vi "Lab Panel V4.88.vi"() -> ()   [LabVIEW 2013] (continued)
                    n2522 = Bundle("FAIL LAB02-2"=w4756, "SIG LAB02-2"=w4766, "TEMP START LAB02-2"=w4765, "DISP LAB02-2"=w4762, "SET LAB02-2"=w4761, "TDMS LAB02-2"=w4764) -> (w4751:T35)  [unwired: 1 in]
                    n2523 = call "sub vi - cycle&temp fail v7.vi"("Amps Lo?"=w4763, "Input Cluster"=w4751, "SELECT"=w4760, "Amps Hi?"=w4759, "Result In"=w4753) -> ("(FAIL) out"=w4755:cluster{"FAIL LO":dbl, "FAIL HI":dbl}, "(DISP) out"=w4758:T4, "T-RISE"=w4752:cluster{"T-RISE (L)":dbl, "T-RISE (N)":dbl}, "Result Out"=w4754:bool, "file error"=w4757:errorcluster)  [unwired: 10 in]
                    n2524 = local write "TEMP RISE LAB02-2"(w4752) -> ()
                    n2525 = local write "FAIL LAB02-2"(w4755) -> ()
                    n2526 = local write "DISP LAB02-2"(w4758) -> ()
                    n2527 = local write "RESULT LAB02-2"(w4754) -> ()
                    n2528 = local write "data file error"(w4757) -> ()
                  }
                }
              }
              frame #4 {
                # "LAB03-1"
                n2529 = case shown="True" w4768 {
                  tunnel: w4770 -> [_ w4783]
                  tunnel: w4767 -> [_ w4780]
                  tunnel: w4769 -> [_ w4779]
                  frame False {
                  }
                  frame True {
                    n2530 = local read "TEMP START LAB03-1"() -> (w4785:cluster{"TL":dbl, "TN":dbl})
                    n2531 = local read "FAIL LAB03-1"() -> (w4776:cluster{"LO":dbl, "HI":dbl})
                    n2532 = local read "TDMS LAB03-1"() -> (w4784:refnum<k34>)
                    n2533 = local read "SET LAB03-1"() -> (w4781:T5)
                    n2534 = local read "DISP LAB03-1"() -> (w4782:T4)
                    n2535 = local read "SIG LAB03-1"() -> (w4786:T2)
                    n2536 = local read "RESULT LAB03-1"() -> (w4773:bool)
                    n2537 = Bundle("FAIL LAB03-1"=w4776, "SIG LAB03-1"=w4786, "TEMP START LAB03-1"=w4785, "DISP LAB03-1"=w4782, "SET LAB03-1"=w4781, "TDMS LAB03-1"=w4784) -> (w4771:T36)  [unwired: 1 in]
                    n2538 = call "sub vi - cycle&temp fail v7.vi"("Amps Lo?"=w4783, "Input Cluster"=w4771, "SELECT"=w4780, "Amps Hi?"=w4779, "Result In"=w4773) -> ("(FAIL) out"=w4775:cluster{"FAIL LO":dbl, "FAIL HI":dbl}, "(DISP) out"=w4778:T4, "T-RISE"=w4772:cluster{"T-RISE (L)":dbl, "T-RISE (N)":dbl}, "Result Out"=w4774:bool, "file error"=w4777:errorcluster)  [unwired: 10 in]
                    n2539 = local write "TEMP RISE LAB03-1"(w4772) -> ()
                    n2540 = local write "FAIL LAB03-1"(w4775) -> ()
                    n2541 = local write "DISP LAB03-1"(w4778) -> ()
                    n2542 = local write "RESULT LAB03-1"(w4774) -> ()
                    n2543 = local write "data file error"(w4777) -> ()
                  }
                }
              }
              frame #5 {
                # "LAB03-2"
                n2544 = case shown="True" w4788 {
                  tunnel: w4790 -> [_ w4803]
                  tunnel: w4787 -> [_ w4800]
                  tunnel: w4789 -> [_ w4799]
                  frame False {
                  }
                  frame True {
                    n2545 = local read "TEMP START LAB03-2"() -> (w4805:cluster{"TL":dbl, "TN":dbl})
                    n2546 = local read "FAIL LAB03-2"() -> (w4796:cluster{"LO":dbl, "HI":dbl})
                    n2547 = local read "TDMS LAB03-2"() -> (w4804:refnum<k34>)
                    n2548 = local read "SET LAB03-2"() -> (w4801:T5)
                    n2549 = local read "DISP LAB03-2"() -> (w4802:T4)
                    n2550 = local read "RESULT LAB03-2"() -> (w4793:bool)
                    n2551 = local read "SIG LAB03-2"() -> (w4806:T2)
                    n2552 = Bundle("FAIL LAB03-2"=w4796, "SIG LAB03-2"=w4806, "TEMP START LAB03-2"=w4805, "DISP LAB03-2"=w4802, "SET LAB03-2"=w4801, "TDMS LAB03-2"=w4804) -> (w4791:T37)  [unwired: 1 in]
                    n2553 = call "sub vi - cycle&temp fail v7.vi"("Amps Lo?"=w4803, "Input Cluster"=w4791, "SELECT"=w4800, "Amps Hi?"=w4799, "Result In"=w4793) -> ("(FAIL) out"=w4795:cluster{"FAIL LO":dbl, "FAIL HI":dbl}, "(DISP) out"=w4798:T4, "T-RISE"=w4792:cluster{"T-RISE (L)":dbl, "T-RISE (N)":dbl}, "Result Out"=w4794:bool, "file error"=w4797:errorcluster)  [unwired: 10 in]
                    n2554 = local write "FAIL LAB03-2"(w4795) -> ()
                    n2555 = local write "TEMP RISE LAB03-2"(w4792) -> ()
                    n2556 = local write "DISP LAB03-2"(w4798) -> ()
                    n2557 = local write "RESULT LAB03-2"(w4794) -> ()
                    n2558 = local write "data file error"(w4797) -> ()
                  }
                }
              }
              frame #6 {
                # "LAB04-1"
                n2559 = case shown="True" w4808 {
                  tunnel: w4810 -> [_ w4823]
                  tunnel: w4807 -> [_ w4820]
                  tunnel: w4809 -> [_ w4819]
                  frame False {
                  }
                  frame True {
                    n2560 = local read "TEMP START LAB04-1"() -> (w4825:cluster{"TL":dbl, "TN":dbl})
                    n2561 = local read "FAIL LAB04-1"() -> (w4816:cluster{"LO":dbl, "HI":dbl})
                    n2562 = local read "TDMS LAB04-1"() -> (w4824:refnum<k34>)
                    n2563 = local read "SET LAB04-1"() -> (w4821:T5)
                    n2564 = local read "DISP LAB04-1"() -> (w4822:T4)
                    n2565 = local read "SIG LAB04-1"() -> (w4826:T2)
                    n2566 = local read "RESULT LAB04-1"() -> (w4813:bool)
                    n2567 = Bundle("FAIL LAB04-1"=w4816, "SIG LAB04-1"=w4826, "TEMP START LAB04-1"=w4825, "DISP LAB04-1"=w4822, "SET LAB04-1"=w4821, "TDMS LAB04-1"=w4824) -> (w4811:T38)  [unwired: 1 in]
                    n2568 = call "sub vi - cycle&temp fail v7.vi"("Amps Lo?"=w4823, "Input Cluster"=w4811, "SELECT"=w4820, "Amps Hi?"=w4819, "Result In"=w4813) -> ("(FAIL) out"=w4815:cluster{"FAIL LO":dbl, "FAIL HI":dbl}, "(DISP) out"=w4818:T4, "T-RISE"=w4812:cluster{"T-RISE (L)":dbl, "T-RISE (N)":dbl}, "Result Out"=w4814:bool, "file error"=w4817:errorcluster)  [unwired: 10 in]
                    n2569 = local write "TEMP RISE LAB04-1"(w4812) -> ()
                    n2570 = local write "FAIL LAB04-1"(w4815) -> ()
                    n2571 = local write "DISP LAB04-1"(w4818) -> ()
                    n2572 = local write "RESULT LAB04-1"(w4814) -> ()
                    n2573 = local write "data file error"(w4817) -> ()
                  }
                }
              }
              frame #7 {
                # "LAB04-2"
                n2574 = case shown="True" w4828 {
                  tunnel: w4830 -> [_ w4843]
                  tunnel: w4827 -> [_ w4840]
                  tunnel: w4829 -> [_ w4839]
                  frame False {
                  }
                  frame True {
                    n2575 = local read "TEMP START LAB04-2"() -> (w4845:cluster{"TL":dbl, "TN":dbl})
                    n2576 = local read "FAIL LAB04-2"() -> (w4836:cluster{"LO":dbl, "HI":dbl})
                    n2577 = local read "TDMS LAB04-2"() -> (w4844:refnum<k34>)
                    n2578 = local read "SET LAB04-2"() -> (w4841:T5)
                    n2579 = local read "DISP LAB04-2"() -> (w4842:T4)
                    n2580 = local read "SIG LAB04-2"() -> (w4846:T2)
                    n2581 = local read "RESULT LAB04-2"() -> (w4833:bool)
                    n2582 = Bundle("FAIL LAB04-2"=w4836, "SIG LAB04-2"=w4846, "TEMP START LAB04-2"=w4845, "DISP LAB04-2"=w4842, "SET LAB04-2"=w4841, "TDMS LAB04-2"=w4844) -> (w4831:T39)  [unwired: 1 in]
                    n2583 = call "sub vi - cycle&temp fail v7.vi"("Amps Lo?"=w4843, "Input Cluster"=w4831, "SELECT"=w4840, "Amps Hi?"=w4839, "Result In"=w4833) -> ("(FAIL) out"=w4835:cluster{"FAIL LO":dbl, "FAIL HI":dbl}, "(DISP) out"=w4838:T4, "T-RISE"=w4832:cluster{"T-RISE (L)":dbl, "T-RISE (N)":dbl}, "Result Out"=w4834:bool, "file error"=w4837:errorcluster)  [unwired: 10 in]
                    n2584 = local write "TEMP RISE LAB04-2"(w4832) -> ()
                    n2585 = local write "FAIL LAB04-2"(w4835) -> ()
                    n2586 = local write "DISP LAB04-2"(w4838) -> ()
                    n2587 = local write "RESULT LAB04-2"(w4834) -> ()
                    n2588 = local write "data file error"(w4837) -> ()
                  }
                }
              }
              frame #8 {
                # "LAB05-1"
                n2589 = case shown="True" w4848 {
                  tunnel: w4850 -> [_ w4863]
                  tunnel: w4847 -> [_ w4860]
                  tunnel: w4849 -> [_ w4859]
                  frame False {
                  }
                  frame True {
                    n2590 = local read "TEMP START LAB05-1"() -> (w4865:cluster{"TL":dbl, "TN":dbl})
                    n2591 = local read "FAIL LAB05-1"() -> (w4856:cluster{"LO":dbl, "HI":dbl})
                    n2592 = local read "TDMS LAB05-1"() -> (w4864:refnum<k34>)
                    n2593 = local read "SET LAB05-1"() -> (w4861:T5)
                    n2594 = local read "DISP LAB05-1"() -> (w4862:T4)
                    n2595 = local read "SIG LAB05-1"() -> (w4866:T2)
                    n2596 = local read "RESULT LAB05-1"() -> (w4853:bool)
                    n2597 = Bundle("FAIL LAB05-1"=w4856, "SIG LAB05-1"=w4866, "TEMP START LAB05-1"=w4865, "DISP LAB05-1"=w4862, "SET LAB05-1"=w4861, "TDMS LAB05-1"=w4864) -> (w4851:T40)  [unwired: 1 in]
                    n2598 = call "sub vi - cycle&temp fail v7.vi"("Amps Lo?"=w4863, "Input Cluster"=w4851, "SELECT"=w4860, "Amps Hi?"=w4859, "Result In"=w4853) -> ("(FAIL) out"=w4855:cluster{"FAIL LO":dbl, "FAIL HI":dbl}, "(DISP) out"=w4858:T4, "T-RISE"=w4852:cluster{"T-RISE (L)":dbl, "T-RISE (N)":dbl}, "Result Out"=w4854:bool, "file error"=w4857:errorcluster)  [unwired: 10 in]
                    n2599 = local write "TEMP RISE LAB05-1"(w4852) -> ()
                    n2600 = local write "FAIL LAB05-1"(w4855) -> ()
                    n2601 = local write "DISP LAB05-1"(w4858) -> ()
                    n2602 = local write "RESULT LAB05-1"(w4854) -> ()
                    n2603 = local write "data file error"(w4857) -> ()
                  }
                }
              }
              frame #9 {
                # "LAB05-2"
                n2604 = case shown="True" w4868 {
                  tunnel: w4870 -> [_ w4883]
                  tunnel: w4867 -> [_ w4880]
                  tunnel: w4869 -> [_ w4879]
                  frame False {
                  }
                  frame True {
                    n2605 = local read "TEMP START LAB05-2"() -> (w4885:cluster{"TL":dbl, "TN":dbl})
                    n2606 = local read "FAIL LAB05-2"() -> (w4876:cluster{"LO":dbl, "HI":dbl})
                    n2607 = local read "TDMS LAB05-2"() -> (w4884:refnum<k34>)
                    n2608 = local read "SET LAB05-2"() -> (w4881:T5)
                    n2609 = local read "DISP LAB05-2"() -> (w4882:T4)
                    n2610 = local read "SIG LAB05-2"() -> (w4886:T2)
                    n2611 = local read "RESULT LAB05-2"() -> (w4873:bool)
                    n2612 = Bundle("FAIL LAB05-2"=w4876, "SIG LAB05-2"=w4886, "TEMP START LAB05-2"=w4885, "DISP LAB05-2"=w4882, "SET LAB05-2"=w4881, "TDMS LAB05-2"=w4884) -> (w4871:T41)  [unwired: 1 in]
                    n2613 = call "sub vi - cycle&temp fail v7.vi"("Amps Lo?"=w4883, "Input Cluster"=w4871, "SELECT"=w4880, "Amps Hi?"=w4879, "Result In"=w4873) -> ("(FAIL) out"=w4875:cluster{"FAIL LO":dbl, "FAIL HI":dbl}, "(DISP) out"=w4878:T4, "T-RISE"=w4872:cluster{"T-RISE (L)":dbl, "T-RISE (N)":dbl}, "Result Out"=w4874:bool, "file error"=w4877:errorcluster)  [unwired: 10 in]
                    n2614 = local write "TEMP RISE LAB05-2"(w4872) -> ()
                    n2615 = local write "FAIL LAB05-2"(w4875) -> ()
                    n2616 = local write "DISP LAB05-2"(w4878) -> ()
                    n2617 = local write "RESULT LAB05-2"(w4874) -> ()
                    n2618 = local write "data file error"(w4877) -> ()
                  }
                }
              }
            }
          }
          frame #15 {
            # "run calibration routine"
            n2619 = local read "SET (cal)"() -> (w4887:bool)
            n2620 = case shown="True" w4887 {
              frame False {
              }
              frame True {
                n2621 = stacked-sequence {
                  seq-local: [w4888 _ _] -> [_ w4890 _]
                  frame #0 {
                    n2622 = call "CALIBRATION PASSWORD"() -> ("PASSWORD"=w4888:string)  [unwired: 17 in, 2 out]
                  }
                  frame #1 {
                    n2623 = Equal?(x=w4890, y="7777") -> (x = y?=w4889:bool)
                    n2624 = case shown="True" w4889 {
                      frame False {
                      }
                      frame True {
                        n2625 = stacked-sequence {
                          frame #0 {
                            n2626 = local read "Temp Test Cal"() -> (w4892:dbl)
                            n2627 = call "sub vi - calibration v1.vi"("Temp Test Cal"=w4892) -> ()  [unwired: 11 in]
                          }
                          frame #1 {
                            n2628 = call "sub vi - get calibration values v1.vi"() -> ("TEMP REF CAL"=w4893:dbl, "LAB01 (CAL)"=w4898:T14, "LAB02 (CAL)"=w4897:T15, "LAB03 (CAL)"=w4896:T14, "LAB04 (CAL)"=w4895:T14, "calibration file error out"=w4899:errorcluster, "LAB05 (CAL)"=w4894:T14)  [unwired: 9 in]
                            n2629 = local write "TEMP REF cal"(w4893) -> ()
                            n2630 = local write "cal file error out"(w4899) -> ()
                            n2631 = local write "CAL LAB04"(w4895) -> ()
                            n2632 = local write "CAL LAB05"(w4894) -> ()
                            n2633 = local write "CAL LAB01"(w4898) -> ()
                            n2634 = local write "CAL LAB02"(w4897) -> ()
                            n2635 = local write "CAL LAB03"(w4896) -> ()
                          }
                        }
                      }
                    }
                  }
                  frame #2 {
                    n2636 = local write "SET (cal)"(FALSE) -> ()
                  }
                }
              }
            }
          }
          frame #16 {
            # "save certain settings to file"
            n2637 = String To Path(string="c:\\crabtree\\Set Up\\") -> (path=w4902:path)
            n2638 = Build Path(base path=w4902, name or relative path="settings.bin") -> (appended path=w4904:path)
            n2639 = Build Path(base path=w4902, name or relative path="mail.bin") -> (appended path=w4901:path)
            n2640 = Create Folder(path (use dialog)=w4902) -> (error out=w4907:errorcluster)  [unwired: 2 in, 2 out]
            n2641 = call <vilib>:"Clear Errors.vi"("error in (no error)"=w4907) -> ()  [unwired: 6 in, 1 out]
            n2642 = stacked-sequence {
              seq-local: [w4919 _] -> [_ w4932]
              tunnel: w4904 -> [_ w4933]
              tunnel: w4901 -> [_ w4931]
              frame #0 {
                n2643 = local read "C drive data root dir"() -> (w4918:path)
                n2644 = local read "Select COM port"() -> (w4915:refnum<visa-resource-name>)
                n2645 = local read "Network Directory"() -> (w4924:path)
                n2646 = local read "SET LAB05-2"() -> (w4923:T5)
                n2647 = local read "SET LAB05-1"() -> (w4922:T5)
                n2648 = local read "SET LAB04-2"() -> (w4921:T5)
                n2649 = local read "SET LAB03-2"() -> (w4925:T5)
                n2650 = local read "SET LAB04-1"() -> (w4920:T5)
                n2651 = local read "SET LAB03-1"() -> (w4926:T5)
                n2652 = local read "SET LAB02-2"() -> (w4927:T5)
                n2653 = local read "SET LAB02-1"() -> (w4928:T5)
                n2654 = local read "Temp Delay Lps"() -> (w4914:dbl)
                n2655 = local read "Amps Fail level"() -> (w4910:dbl)
                n2656 = local read "SET LAB01-2"() -> (w4929:T5)
                n2657 = local read "Temp Test Cal"() -> (w4911:dbl)
                n2658 = local read "SET LAB01-1"() -> (w4930:T5)
                n2659 = local read "Mail Test File To:"() -> (w4909:string)
                n2660 = local read "Temp Value"() -> (w4913:dbl)
                n2661 = local read "Fail Loops"() -> (w4912:dbl)
                n2662 = local read "Mail Test Fail"() -> (w4908:bool)
                n2663 = local read "RATE (Hz)"() -> (w4917:dbl)
                n2664 = local read "SAMPLES"() -> (w4916:dbl)
                n2665 = Bundle("SET LAB01-1"=w4930, "SET LAB01-2"=w4929, "SET LAB02-1"=w4928, "SET LAB02-2"=w4927, "SET LAB03-1"=w4926, "SET LAB03-2"=w4925, "SET LAB04-1"=w4920, "SET LAB04-2"=w4921, "SET LAB05-1"=w4922, "SET LAB05-2"=w4923, "Network Directory"=w4924, "C drive data root dir"=w4918, "RATE (Hz)"=w4917, "SAMPLES"=w4916, "Select COM port"=w4915, "Temp Delay Lps"=w4914, "Temp Value"=w4913, "Fail Loops"=w4912, "Temp Test Cal"=w4911, "Amps Fail level"=w4910, "Mail Test File To:"=w4909, "Mail Test Fail"=w4908) -> (w4919:T22)  [unwired: 1 in]
              }
              frame #1 {
                n2666 = event shown="[1] \"SET LAB01-1\", \"SET LAB01-2\", \"SET LAB02-1\", \"SET LAB02-2\", \"SET LAB03-1\", \"SET LAB03-2\", \"SET LAB04-1\", \"SET LAB04-2\", \"SET LAB05-1\", \"SET LAB05-2\", \"Network Directory\", \"C drive data root dir\", \"RATE (Hz)\", \"SAMPLES\", \"Select COM port\", \"Temp Delay Lps\", \"Temp Value\", \"Fail Loops\", \"Temp Test Cal\", \"Amps Fail level\", \"Mail Test File To:\", \"Mail Test Fail\": Value Change" {
                  selector: _ -> [_ _ _]
                  dyn-events: _ -> [_ _ _]
                  timeout: 10.0 -> [_ _ _]
                  tunnel: w4933 -> [_ w4935 _]
                  tunnel: w4932 -> [_ w4936 _]
                  tunnel: w4931 -> [_ _ w4947]
                  event Timeout {
                    n2667 = event-data() -> ()  [unwired: 1 in, 3 out]
                  }
                  event "SET LAB01-1", "SET LAB01-2", "SET LAB02-1", "SET LAB02-2", "SET LAB03-1", "SET LAB03-2", "SET LAB04-1", "SET LAB04-2", "SET LAB05-1", "SET LAB05-2", "Network Directory", "C drive data root dir", "RATE (Hz)", "SAMPLES", "Select COM port", "Temp Delay Lps", "Temp Value", "Fail Loops", "Temp Test Cal", "Amps Fail level", "Mail Test File To:", "Mail Test Fail": Value Change {
                    n2668 = event-data() -> ()  [unwired: 1 in, 6 out]
                    n2669 = Open/Create/Replace File(file path (use dialog)=w4935, operation (0:open)=T21."replace or create") -> (refnum out=w4941:refnum<file>, error out=w4940:errorcluster)  [unwired: 4 in, 1 out]
                    n2670 = Write to Binary File(file (use dialog)=w4941, data=w4936, error in=w4940) -> (refnum out=w4939:refnum<file>, error out=w4938:errorcluster)  [unwired: 3 in, 1 out]
                    n2671 = Close File(refnum=w4939, error in=w4938) -> (error out=w4937:errorcluster)  [unwired: 1 out]
                    n2672 = local write "data file error"(w4937) -> ()
                  }
                  event "MAIL SETTINGS.OUT SERVER ADDRESS", "MAIL SETTINGS.FROM ACCOUNT", "MAIL SETTINGS.USER NAME", "MAIL SETTINGS.PASSWORD", "Auto Mail Send", "TO (string):": Value Change {
                    n2673 = event-data() -> ()  [unwired: 1 in, 6 out]
                    n2674 = local read "MAIL SETTINGS"() -> (w4946:T7)
                    n2675 = local read "Auto Mail Send"() -> (w4944:bool)
                    n2676 = local read "TO (string):"() -> (w4943:string)
                    n2677 = Open/Create/Replace File(file path (use dialog)=w4947, operation (0:open)=T21."replace or create") -> (refnum out=w4952:refnum<file>, error out=w4951:errorcluster)  [unwired: 4 in, 1 out]
                    n2678 = Bundle("MAIL SETTINGS"=w4946, "Auto Mail Send"=w4944, "TO (string):"=w4943) -> (w4945:T42)  [unwired: 1 in]
                    n2679 = Write to Binary File(file (use dialog)=w4952, data=w4945, error in=w4951) -> (refnum out=w4950:refnum<file>, error out=w4949:errorcluster)  [unwired: 3 in, 1 out]
                    n2680 = Close File(refnum=w4950, error in=w4949) -> (error out=w4948:errorcluster)  [unwired: 1 out]
                    n2681 = local write "data file error"(w4948) -> ()
                  }
                }
              }
            }
          }
          frame #17 {
            # "mail control"
            n2682 = local read "MAIL SETTINGS"() -> (w4969:T7)
            n2683 = local read "Auto Mail Send"() -> (w4955:bool)
            n2684 = Unbundle(w4969) -> ("OUT SERVER ADDRESS"=w4968:string, "FROM ACCOUNT"=w4967:string, "TEST MAIL"=w4966:bool)  [unwired: 4 out]
            n2685 = stacked-sequence {
              tunnel: "TO (string):" -> [_ w5008]
              tunnel: w4969 -> [w4974 w5007]
              tunnel: w4968 -> [w4973 w5006]
              tunnel: w4967 -> [w4972 w5005]
              tunnel: w4966 -> [w4971 _]
              tunnel: w4955 -> [_ w5004]
              tunnel: w4965 -> [_ w5003]
              tunnel: w4964 -> [_ w5002]
              tunnel: w4963 -> [_ w5001]
              tunnel: w4962 -> [_ w5000]
              tunnel: w4961 -> [_ w4999]
              tunnel: w4960 -> [_ w4998]
              tunnel: w4959 -> [_ w4997]
              tunnel: w4958 -> [_ w4996]
              tunnel: w4957 -> [_ w4995]
              tunnel: w4956 -> [_ w4994]
              tunnel: "TO (string):" -> [w4970 _]
              frame #0 {
                # "mail test"
                n2686 = case shown="True" w4971 {
                  tunnel: w4974 -> [_ w4978]
                  tunnel: w4970 -> [_ w4977]
                  tunnel: w4973 -> [_ w4976]
                  tunnel: w4972 -> [_ w4975]
                  frame False {
                  }
                  frame True {
                    n2687 = stacked-sequence {
                      seq-local: [_ _ w4988 _] -> [_ _ _ w4989]
                      tunnel: w4978 -> [w4981 _ _ w4993]
                      tunnel: w4977 -> [_ _ w4986 _]
                      tunnel: w4976 -> [_ _ w4984 _]
                      tunnel: w4975 -> [_ _ w4985 _]
                      frame #0 {
                        n2688 = Bundle(cluster=w4981, "TEST MAIL STATUS"="TEST START") -> (w4979:T7)  [unwired: 6 in]
                        n2689 = local write "MAIL SETTINGS"(w4979) -> ()
                      }
                      frame #1 {
                        n2690 = Wait (ms)(milliseconds to wait=500) -> ()  [unwired: 1 out]
                      }
                      frame #2 {
                        n2691 = call "sub vi - send mail v5.vi"("TO:"=w4986, "subject"="MAIL TEST FROM LAB PANEL", "from"=w4985, "out going server"=w4984, "message"="TEST MESSAGE") -> ("error out"=w4988:errorcluster)  [unwired: 10 in]
                      }
                      frame #3 {
                        n2692 = Bundle(cluster=w4993, "TEST MAIL"=FALSE, "TEST MAIL STATUS"="TEST END", "mail error"=w4989) -> (w4991:T7)  [unwired: 4 in]
                        n2693 = local write "MAIL SETTINGS"(w4991) -> ()
                      }
                    }
                  }
                }
              }
              frame #1 {
                # "mail report"
                n2694 = stacked-sequence {
                  seq-local: [_ w5051 _ _] -> [_ _ _ w5241]
                  seq-local: [_ _ w5154 _] -> [_ _ _ w5231]
                  seq-local: [w5018 _ _ _] -> [_ w5068 _ _]
                  seq-local: [w5017 _ _ _] -> [_ w5067 _ _]
                  seq-local: [w5015 _ _ _] -> [_ w5065 _ _]
                  seq-local: [w5016 _ _ _] -> [_ w5066 _ _]
                  seq-local: [w5014 _ _ _] -> [_ w5064 _ _]
                  seq-local: [w5013 _ _ _] -> [_ w5059 _ _]
                  seq-local: [w5012 _ _ _] -> [_ w5060 _ _]
                  seq-local: [w5011 _ _ _] -> [_ w5061 _ _]
                  seq-local: [w5010 _ _ _] -> [_ w5062 _ _]
                  seq-local: [w5009 _ _ _] -> [_ w5063 _ _]
                  tunnel: w5008 -> [_ _ _ w5242]
                  tunnel: w5007 -> [_ _ _ w5225]
                  tunnel: w5006 -> [_ _ _ w5239]
                  tunnel: w5005 -> [_ _ _ w5238]
                  tunnel: w5004 -> [w5049 _ _ w5233]
                  tunnel: w5003 -> [_ _ w5184 _]
                  tunnel: w5002 -> [_ _ w5181 _]
                  tunnel: w5001 -> [_ _ w5180 _]
                  tunnel: w5000 -> [_ _ w5179 _]
                  tunnel: w4999 -> [_ _ w5178 _]
                  tunnel: w4998 -> [_ _ w5177 _]
                  tunnel: w4997 -> [_ _ w5176 _]
                  tunnel: w4996 -> [_ _ w5175 _]
                  tunnel: w4995 -> [_ _ w5174 _]
                  tunnel: w4994 -> [_ _ w5173 _]
                  frame #0 {
                    n2695 = case shown="False" w5049 {
                      frame False {
                        n2696 = local write "mail control"("") -> ()
                      }
                      frame True {
                      }
                    }
                    n2697 = local read "SET LAB01-1"() -> (w5048:T5)
                    n2698 = local read "SET LAB01-2"() -> (w5047:T5)
                    n2699 = local read "SET LAB02-1"() -> (w5046:T5)
                    n2700 = local read "SET LAB02-2"() -> (w5045:T5)
                    n2701 = local read "SET LAB03-1"() -> (w5044:T5)
                    n2702 = local read "SET LAB04-1"() -> (w5042:T5)
                    n2703 = local read "SET LAB05-1"() -> (w5040:T5)
                    n2704 = local read "SET LAB03-2"() -> (w5043:T5)
                    n2705 = local read "SET LAB04-2"() -> (w5041:T5)
                    n2706 = local read "SET LAB05-2"() -> (w5039:T5)
                    n2707 = Unbundle(w5044) -> ("DESCRIPTION"=w5024:string)  [unwired: 4 out]
                    n2708 = Unbundle(w5043) -> ("DESCRIPTION"=w5023:string)  [unwired: 4 out]
                    n2709 = Unbundle(w5042) -> ("DESCRIPTION"=w5022:string)  [unwired: 4 out]
                    n2710 = Unbundle(w5039) -> ("DESCRIPTION"=w5019:string)  [unwired: 4 out]
                    n2711 = Unbundle(w5045) -> ("DESCRIPTION"=w5025:string)  [unwired: 4 out]
                    n2712 = Unbundle(w5041) -> ("DESCRIPTION"=w5021:string)  [unwired: 4 out]
                    n2713 = Unbundle(w5048) -> ("DESCRIPTION"=w5037:string)  [unwired: 4 out]
                    n2714 = Unbundle(w5046) -> ("DESCRIPTION"=w5026:string)  [unwired: 4 out]
                    n2715 = Unbundle(w5040) -> ("DESCRIPTION"=w5020:string)  [unwired: 4 out]
                    n2716 = Unbundle(w5047) -> ("DESCRIPTION"=w5027:string)  [unwired: 4 out]
                    n2717 = Concatenate Strings("[LAB05-2/", w5019) -> (w5009:string)
                    n2718 = Concatenate Strings("[LAB05-1/", w5020) -> (w5010:string)
                    n2719 = Concatenate Strings("[LAB04-2/", w5021) -> (w5011:string)
                    n2720 = Concatenate Strings("[LAB03-2/", w5023) -> (w5013:string)
                    n2721 = Concatenate Strings("[LAB04-1/", w5022) -> (w5012:string)
                    n2722 = Concatenate Strings("[LAB03-1/", w5024) -> (w5014:string)
                    n2723 = Concatenate Strings("[LAB01-2/", w5027) -> (w5017:string)
                    n2724 = Concatenate Strings("[LAB02-2/", w5025) -> (w5015:string)
                    n2725 = Concatenate Strings("[LAB01-1/", w5037) -> (w5018:string)
                    n2726 = Concatenate Strings("[LAB02-1/", w5026) -> (w5016:string)
                  }
                  frame #1 {
                    w5072 = "/"
                    w5073 = 2.0
                    n2727 = local read "DISP LAB01-2"() -> (w5152:T4)
                    n2728 = local read "DISP LAB01-1"() -> (w5153:T4)
                    n2729 = local read "DISP LAB02-1"() -> (w5151:T4)
                    n2730 = local read "DISP LAB03-2"() -> (w5148:T4)
                    n2731 = local read "DISP LAB02-2"() -> (w5150:T4)
                    n2732 = local read "DISP LAB03-1"() -> (w5149:T4)
                    n2733 = local read "DISP LAB04-2"() -> (w5146:T4)
                    n2734 = local read "DISP LAB04-1"() -> (w5147:T4)
                    n2735 = local read "DISP LAB05-1"() -> (w5145:T4)
                    n2736 = local read "DISP LAB05-2"() -> (w5144:T4)
                    n2737 = Unbundle(w5152) -> ("CYCLE"=w5136:dbl, "MINS"=w5135:dbl, "STATUS"=w5132:string)
                    n2738 = Unbundle(w5153) -> ("CYCLE"=w5141:dbl, "MINS"=w5140:dbl, "STATUS"=w5137:string)
                    n2739 = Unbundle(w5151) -> ("CYCLE"=w5129:dbl, "MINS"=w5128:dbl, "STATUS"=w5127:string)
                    n2740 = Unbundle(w5148) -> ("CYCLE"=w5116:dbl, "MINS"=w5115:dbl, "STATUS"=w5112:string)
                    n2741 = Unbundle(w5149) -> ("CYCLE"=w5121:dbl, "MINS"=w5120:dbl, "STATUS"=w5117:string)
                    n2742 = Unbundle(w5150) -> ("CYCLE"=w5126:dbl, "MINS"=w5125:dbl, "STATUS"=w5122:string)
                    n2743 = Unbundle(w5147) -> ("CYCLE"=w5111:dbl, "MINS"=w5110:dbl, "STATUS"=w5107:string)
                    n2744 = Unbundle(w5146) -> ("CYCLE"=w5106:dbl, "MINS"=w5105:dbl, "STATUS"=w5102:string)
                    n2745 = Unbundle(w5145) -> ("CYCLE"=w5101:dbl, "MINS"=w5100:dbl, "STATUS"=w5097:string)
                    n2746 = Unbundle(w5144) -> ("CYCLE"=w5143:dbl, "MINS"=w5142:dbl, "STATUS"=w5094:string)
                    n2747 = Number To Decimal String(number=w5129) -> (decimal integer string=w5131:string)  [unwired: 1 in]
                    n2748 = Number To Decimal String(number=w5126) -> (decimal integer string=w5124:string)  [unwired: 1 in]
                    n2749 = Number To Decimal String(number=w5121) -> (decimal integer string=w5119:string)  [unwired: 1 in]
                    n2750 = Number To Decimal String(number=w5136) -> (decimal integer string=w5134:string)  [unwired: 1 in]
                    n2751 = Number To Decimal String(number=w5116) -> (decimal integer string=w5114:string)  [unwired: 1 in]
                    n2752 = Number To Decimal String(number=w5141) -> (decimal integer string=w5139:string)  [unwired: 1 in]
                    n2753 = Number To Decimal String(number=w5143) -> (decimal integer string=w5096:string)  [unwired: 1 in]
                    n2754 = Number To Decimal String(number=w5111) -> (decimal integer string=w5109:string)  [unwired: 1 in]
                    n2755 = Number To Decimal String(number=w5106) -> (decimal integer string=w5104:string)  [unwired: 1 in]
                    n2756 = Number To Decimal String(number=w5101) -> (decimal integer string=w5099:string)  [unwired: 1 in]
                    n2757 = Number To Fractional String(number=w5128, precision (6)=w5073) -> (F-format string=w5130:string)  [unwired: 2 in]
                    n2758 = Number To Fractional String(number=w5115, precision (6)=w5073) -> (F-format string=w5113:string)  [unwired: 2 in]
                    n2759 = Number To Fractional String(number=w5125, precision (6)=w5073) -> (F-format string=w5123:string)  [unwired: 2 in]
                    n2760 = Number To Fractional String(number=w5120, precision (6)=w5073) -> (F-format string=w5118:string)  [unwired: 2 in]
                    n2761 = Number To Fractional String(number=w5105, precision (6)=w5073) -> (F-format string=w5103:string)  [unwired: 2 in]
                    n2762 = Number To Fractional String(number=w5110, precision (6)=w5073) -> (F-format string=w5108:string)  [unwired: 2 in]
                    n2763 = Number To Fractional String(number=w5135, precision (6)=w5073) -> (F-format string=w5133:string)  [unwired: 2 in]
                    n2764 = Number To Fractional String(number=w5100, precision (6)=w5073) -> (F-format string=w5098:string)  [unwired: 2 in]
                    n2765 = Number To Fractional String(number=w5140, precision (6)=w5073) -> (F-format string=w5138:string)  [unwired: 2 in]
                    n2766 = Number To Fractional String(number=w5142, precision (6)=w5073) -> (F-format string=w5095:string)  [unwired: 2 in]
                    n2767 = Concatenate Strings(w5072, w5114, w5072, w5113, w5072, w5112) -> (w5088:string)
                    n2768 = Concatenate Strings(w5072, w5109, w5072, w5108, w5072, w5107) -> (w5087:string)
                    n2769 = Concatenate Strings(w5072, w5104, w5072, w5103, w5072, w5102) -> (w5086:string)
                    n2770 = Concatenate Strings(w5072, w5099, w5072, w5098, w5072, w5097) -> (w5085:string)
                    n2771 = Concatenate Strings(w5072, w5096, w5072, w5095, w5072, w5094) -> (w5084:string)
                    n2772 = Concatenate Strings(w5072, w5139, w5072, w5138, w5072, w5137) -> (w5093:string)
                    n2773 = Concatenate Strings(w5072, w5119, w5072, w5118, w5072, w5117) -> (w5089:string)
                    n2774 = Concatenate Strings(w5072, w5134, w5072, w5133, w5072, w5132) -> (w5092:string)
                    n2775 = Concatenate Strings(w5072, w5131, w5072, w5130, w5072, w5127) -> (w5091:string)
                    n2776 = Concatenate Strings(w5072, w5124, w5072, w5123, w5072, w5122) -> (w5090:string)
                    n2777 = Concatenate Strings("]", "\r") -> (w5069:string)
                    n2778 = Concatenate Strings(w5064, w5089, w5069) -> (w5079:string)
                    n2779 = Concatenate Strings(w5066, w5091, w5069) -> (w5081:string)
                    n2780 = Concatenate Strings(w5065, w5090, w5069) -> (w5080:string)
                    n2781 = Concatenate Strings(w5061, w5086, w5069) -> (w5076:string)
                    n2782 = Concatenate Strings(w5062, w5085, w5069) -> (w5077:string)
                    n2783 = Concatenate Strings(w5060, w5087, w5069) -> (w5075:string)
                    n2784 = Concatenate Strings(w5059, w5088, w5069) -> (w5074:string)
                    n2785 = Concatenate Strings(w5063, w5084, w5069) -> (w5078:string)
                    n2786 = Concatenate Strings(w5067, w5092, w5069) -> (w5082:string)
                    n2787 = Concatenate Strings(w5068, w5093, w5069) -> (w5083:string)
                    n2788 = Concatenate Strings(w5083, w5082, w5081, w5080, w5079, w5074, w5075, w5076, w5077, w5078) -> (w5052:string)
                    n2789 = Concatenate Strings("[PANEL/", "DESC/", "CYCLES/", "MINS/", "STATUS]", "\r", w5052) -> (w5051:string)
                    "MAIL REPORT" <- w5051
                    n2790 = global write "Global display 3.vi" "log all"(w5051) -> ()
                  }
                  frame #2 {
                    w5182 = "END"
                    n2791 = local read "mail control"() -> (w5183:string)
                    n2792 = case shown="False" w5178 {
                      tunnel: w5183 -> [w5207 _]
                      tunnel: w5182 -> [w5206 _]
                      tunnel: [w5205 FALSE] -> w5168
                      frame False {
                        n2793 = Equal?(x=w5207, y=w5206) -> (x = y?=w5205:bool)
                      }
                      frame True {
                      }
                    }
                    n2794 = case shown="False" w5184 {
                      tunnel: w5183 -> [w5223 _]
                      tunnel: w5182 -> [w5222 _]
                      tunnel: [w5221 FALSE] -> w5172
                      frame False {
                        n2795 = Equal?(x=w5223, y=w5222) -> (x = y?=w5221:bool)
                      }
                      frame True {
                      }
                    }
                    n2796 = case shown="False" w5181 {
                      tunnel: w5183 -> [w5219 _]
                      tunnel: w5182 -> [w5218 _]
                      tunnel: [w5217 FALSE] -> w5171
                      frame False {
                        n2797 = Equal?(x=w5219, y=w5218) -> (x = y?=w5217:bool)
                      }
                      frame True {
                      }
                    }
                    n2798 = case shown="False" w5179 {
                      tunnel: w5183 -> [w5211 _]
                      tunnel: w5182 -> [w5210 _]
                      tunnel: [w5209 FALSE] -> w5169
                      frame False {
                        n2799 = Equal?(x=w5211, y=w5210) -> (x = y?=w5209:bool)
                      }
                      frame True {
                      }
                    }
                    n2800 = case shown="False" w5180 {
                      tunnel: w5183 -> [w5215 _]
                      tunnel: w5182 -> [w5214 _]
                      tunnel: [w5213 FALSE] -> w5170
                      frame False {
                        n2801 = Equal?(x=w5215, y=w5214) -> (x = y?=w5213:bool)
                      }
                      frame True {
                      }
                    }
                    n2802 = Or(x=w5170, y=w5169) -> (x .or. y?=w5161:bool)
                    n2803 = Or(x=w5172, y=w5171) -> (x .or. y?=w5162:bool)
                    n2804 = Or(x=w5162, y=w5161) -> (x .or. y?=w5157:bool)
                    n2805 = case shown="False" w5174 {
                      tunnel: w5183 -> [w5191 _]
                      tunnel: w5182 -> [w5190 _]
                      tunnel: [w5189 FALSE] -> w5163
                      frame False {
                        n2806 = Equal?(x=w5191, y=w5190) -> (x = y?=w5189:bool)
                      }
                      frame True {
                      }
                    }
                    n2807 = case shown="False" w5173 {
                      tunnel: w5183 -> [w5187 _]
                      tunnel: w5182 -> [w5186 _]
                      tunnel: [w5185 FALSE] -> w5167
                      frame False {
                        n2808 = Equal?(x=w5187, y=w5186) -> (x = y?=w5185:bool)
                      }
                      frame True {
                      }
                    }
                    n2809 = case shown="False" w5175 {
                      tunnel: w5183 -> [w5195 _]
                      tunnel: w5182 -> [w5194 _]
                      tunnel: [w5193 FALSE] -> w5164
                      frame False {
                        n2810 = Equal?(x=w5195, y=w5194) -> (x = y?=w5193:bool)
                      }
                      frame True {
                      }
                    }
                    n2811 = case shown="False" w5177 {
                      tunnel: w5183 -> [w5203 _]
                      tunnel: w5182 -> [w5202 _]
                      tunnel: [w5201 FALSE] -> w5166
                      frame False {
                        n2812 = Equal?(x=w5203, y=w5202) -> (x = y?=w5201:bool)
                      }
                      frame True {
                      }
                    }
                    n2813 = case shown="False" w5176 {
                      tunnel: w5183 -> [w5199 _]
                      tunnel: w5182 -> [w5198 _]
                      tunnel: [w5197 FALSE] -> w5165
                      frame False {
                        n2814 = Equal?(x=w5199, y=w5198) -> (x = y?=w5197:bool)
                      }
                      frame True {
                      }
                    }
                    n2815 = Or(x=w5166, y=w5165) -> (x .or. y?=w5160:bool)
                    n2816 = Or(x=w5164, y=w5163) -> (x .or. y?=w5159:bool)
                    n2817 = Or(x=w5167, y=w5168) -> (x .or. y?=w5155:bool)
                    n2818 = Or(x=w5160, y=w5159) -> (x .or. y?=w5158:bool)
                    n2819 = Or(x=w5157, y=w5158) -> (x .or. y?=w5156:bool)
                    n2820 = Or(x=w5156, y=w5155) -> (x .or. y?=w5154:bool)
                  }
                  frame #3 {
                    n2821 = local read "on loops"() -> (w5237:dbl)
                    n2822 = local read "jig cycle"() -> (w5234:dbl)
                    n2823 = local read "Send Mail Now"() -> (w5228:bool)
                    n2824 = Add(x=w5237, y=3.0) -> (x+y=w5235:dbl)
                    n2825 = Equal?(x=w5234, y=w5235) -> (x = y?=w5229:bool)
                    n2826 = And(x=w5229, y=w5228) -> (x .and. y?=w5227:bool)
                    n2827 = And(x=w5233, y=w5229) -> (x .and. y?=w5232:bool)
                    n2828 = And(x=w5232, y=w5231) -> (x .and. y?=w5230:bool)
                    n2829 = Or(x=w5230, y=w5227) -> (x .or. y?=w5226:bool)
                    n2830 = case shown="True" w5226 {
                      tunnel: w5242 -> [_ w5248]
                      tunnel: w5241 -> [_ w5247]
                      tunnel: "Lab Panel Test Status" -> [_ w5246]
                      tunnel: w5239 -> [_ w5245]
                      tunnel: w5238 -> [_ w5244]
                      tunnel: w5225 -> [_ w5243]
                      frame False {
                      }
                      frame True {
                        n2831 = stacked-sequence {
                          tunnel: w5248 -> [w5256 _]
                          tunnel: w5247 -> [w5255 _]
                          tunnel: w5246 -> [w5254 _]
                          tunnel: w5245 -> [w5253 _]
                          tunnel: w5244 -> [w5252 _]
                          tunnel: w5243 -> [w5251 _]
                          frame #0 {
                            n2832 = call "sub vi - send mail v5.vi"("TO:"=w5256, "subject"=w5254, "from"=w5252, "out going server"=w5253, "message"=w5255) -> ("error out"=w5250:errorcluster)  [unwired: 10 in]
                            n2833 = Bundle(cluster=w5251, "mail error"=w5250) -> (w5249:T7)  [unwired: 6 in]
                            n2834 = local write "MAIL SETTINGS"(w5249) -> ()
                          }
                          frame #1 {
                            n2835 = local write "mail control"("") -> ()
                            n2836 = local write "Send Mail Now"(FALSE) -> ()
                          }
                        }
                      }
                    }
                  }
                }
              }
            }
          }
          frame #18 {
            # "save jig cycle values once all run switches are off"
            n2837 = stacked-sequence {
              tunnel: w5268 -> [_ w5297]
              tunnel: w5267 -> [_ w5296]
              tunnel: w5266 -> [_ w5295]
              tunnel: w5265 -> [_ w5294]
              tunnel: w5264 -> [_ w5293]
              tunnel: w5263 -> [_ w5292]
              tunnel: w5262 -> [_ w5291]
              tunnel: w5261 -> [_ w5290]
              tunnel: w5260 -> [_ w5289]
              tunnel: w5259 -> [_ w5288]
              frame #0 {
              }
              frame #1 {
                n2838 = Not(x=w5288) -> (.not. x?=w5271:bool)
                n2839 = Not(x=w5296) -> (.not. x?=w5286:bool)
                n2840 = Not(x=w5293) -> (.not. x?=w5281:bool)
                n2841 = Not(x=w5291) -> (.not. x?=w5277:bool)
                n2842 = Not(x=w5289) -> (.not. x?=w5273:bool)
                n2843 = Not(x=w5297) -> (.not. x?=w5287:bool)
                n2844 = Not(x=w5295) -> (.not. x?=w5285:bool)
                n2845 = Not(x=w5292) -> (.not. x?=w5279:bool)
                n2846 = Not(x=w5294) -> (.not. x?=w5283:bool)
                n2847 = Not(x=w5290) -> (.not. x?=w5275:bool)
                n2848 = local read "Save JC"() -> (w5299:bool)
                n2849 = And(x=w5287, y=w5286) -> (x .and. y?=w5284:bool)
                n2850 = And(x=w5284, y=w5285) -> (x .and. y?=w5282:bool)
                n2851 = And(x=w5282, y=w5283) -> (x .and. y?=w5280:bool)
                n2852 = And(x=w5280, y=w5281) -> (x .and. y?=w5278:bool)
                n2853 = And(x=w5278, y=w5279) -> (x .and. y?=w5276:bool)
                n2854 = And(x=w5276, y=w5277) -> (x .and. y?=w5274:bool)
                n2855 = And(x=w5274, y=w5275) -> (x .and. y?=w5272:bool)
                n2856 = And(x=w5272, y=w5273) -> (x .and. y?=w5270:bool)
                n2857 = And(x=w5270, y=w5271) -> (x .and. y?=w5269:bool)
                n2858 = And(x=w5269, y=w5299) -> (x .and. y?=w5298:bool)
                n2859 = case shown="True" w5298 {
                  tunnel: w5269 -> [w5300 _]
                  frame False {
                    n2860 = case shown="False" w5300 {
                      frame False {
                        n2861 = local write "Save JC"(TRUE) -> ()
                      }
                      frame True {
                      }
                    }
                  }
                  frame True {
                    n2862 = stacked-sequence {
                      frame #0 {
                        n2863 = String To Path(string="c:\\crabtree\\Jig Cycles\\") -> (path=w5312:path)
                        n2864 = Build Path(base path=w5312, name or relative path="jigcycles.bin") -> (appended path=w5310:path)
                        n2865 = Create Folder(path (use dialog)=w5312) -> (error out=w5314:errorcluster)  [unwired: 2 in, 2 out]
                        n2866 = local read "JIG RELAY CYCLES"() -> (w5304:T8)
                        n2867 = call <vilib>:"Clear Errors.vi"("error in (no error)"=w5314) -> ()  [unwired: 6 in, 1 out]
                        n2868 = local write "Save JC"(FALSE) -> ()
                        n2869 = Open/Create/Replace File(file path (use dialog)=w5310, operation (0:open)=T21."replace or create") -> (refnum out=w5308:refnum<file>, error out=w5309:errorcluster)  [unwired: 4 in, 1 out]
                        n2870 = Write to Binary File(file (use dialog)=w5308, data=w5304, error in=w5309) -> (refnum out=w5307:refnum<file>, error out=w5306:errorcluster)  [unwired: 3 in, 1 out]
                        n2871 = Close File(refnum=w5307, error in=w5306) -> (error out=w5305:errorcluster)  [unwired: 1 out]
                        n2872 = local write "data file error"(w5305) -> ()
                      }
                      frame #1 {
                        n2873 = local read "JIG RELAY CYCLES"() -> (w5337:T8)
                        n2874 = Unbundle By Name(w5337) -> ("LAB01-1"=w5332:dbl, "LAB01-2"=w5331:dbl, "LAB02-1"=w5329:dbl, "LAB02-2"=w5328:dbl, "LAB03-1"=w5326:dbl, "LAB03-2"=w5323:dbl, "LAB04-1"=w5322:dbl, "LAB04-2"=w5320:dbl, "LAB05-1"=w5318:dbl, "LAB05-2"=w5316:dbl)
                        n2875 = stacked-sequence {
                          tunnel: w5332 -> [w5340 _ _ _ _ _ _ _ _ _]
                          tunnel: 1000000 -> [w5343 w5353 w5363 w5373 w5383 w5393 w5403 w5413 w5423 w5433]
                          tunnel: [w5341 _ _ _ _ _ _ _ _ _] -> w5335
                          tunnel: "TEST STATION HAS REACHED 1 MILLION CYCLES, REPLACE  CONTROL RELAYS" -> [w5339 w5351 w5361 w5371 w5381 w5391 w5401 w5411 w5421 w5431]
                          tunnel: [_ w5350 _ _ _ _ _ _ _ _] -> w5333
                          tunnel: w5331 -> [_ w5349 _ _ _ _ _ _ _ _]
                          tunnel: [_ _ w5360 _ _ _ _ _ _ _] -> w5330
                          tunnel: w5329 -> [_ _ w5359 _ _ _ _ _ _ _]
                          tunnel: w5328 -> [_ _ _ w5370 _ _ _ _ _ _]
                          tunnel: [_ _ _ w5369 _ _ _ _ _ _] -> w5327
                          tunnel: w5326 -> [_ _ _ _ w5380 _ _ _ _ _]
                          tunnel: [_ _ _ _ w5379 _ _ _ _ _] -> w5325
                          tunnel: [_ _ _ _ _ w5390 _ _ _ _] -> w5324
                          tunnel: w5323 -> [_ _ _ _ _ w5389 _ _ _ _]
                          tunnel: w5322 -> [_ _ _ _ _ _ w5400 _ _ _]
                          tunnel: [_ _ _ _ _ _ w5399 _ _ _] -> w5321
                          tunnel: w5320 -> [_ _ _ _ _ _ _ w5410 _ _]
                          tunnel: [_ _ _ _ _ _ _ w5409 _ _] -> w5319
                          tunnel: w5318 -> [_ _ _ _ _ _ _ _ w5420 _]
                          tunnel: [_ _ _ _ _ _ _ _ w5419 _] -> w5317
                          tunnel: w5316 -> [_ _ _ _ _ _ _ _ _ w5430]
                          tunnel: [_ _ _ _ _ _ _ _ _ w5429] -> w5315
                          frame #0 {
                            n2876 = Greater?(x=w5340, y=w5343) -> (0:w5342:bool)
                            n2877 = case shown="True" w5342 {
                              tunnel: [w5344 0] -> w5341
                              tunnel: w5340 -> [w5344 _]
                              tunnel: w5339 -> [_ w5345]
                              frame False {
                              }
                              frame True {
                                n2878 = Concatenate Strings("LA01-1 ", w5345) -> (w5348:string)
                                n2879 = One Button Dialog(message=w5348) -> ()  [unwired: 1 in, 1 out]
                              }
                            }
                          }
                          frame #1 {
                            n2880 = Greater?(x=w5349, y=w5353) -> (0:w5352:bool)
                            n2881 = case shown="True" w5352 {
                              tunnel: [w5354 0] -> w5350
                              tunnel: w5349 -> [w5354 _]
                              tunnel: w5351 -> [_ w5355]
                              frame False {
                              }
                              frame True {
                                n2882 = Concatenate Strings("LA01-2 ", w5355) -> (w5358:string)
                                n2883 = One Button Dialog(message=w5358) -> ()  [unwired: 1 in, 1 out]
                              }
                            }
                          }
                          frame #2 {
                            n2884 = Greater?(x=w5359, y=w5363) -> (0:w5362:bool)
                            n2885 = case shown="True" w5362 {
                              tunnel: [w5364 0] -> w5360
                              tunnel: w5359 -> [w5364 _]
                              tunnel: w5361 -> [_ w5365]
                              frame False {
                              }
                              frame True {
                                n2886 = Concatenate Strings("LA02-1 ", w5365) -> (w5368:string)
                                n2887 = One Button Dialog(message=w5368) -> ()  [unwired: 1 in, 1 out]
                              }
                            }
                          }
                          frame #3 {
                            n2888 = Greater?(x=w5370, y=w5373) -> (0:w5372:bool)
                            n2889 = case shown="True" w5372 {
                              tunnel: [w5374 0] -> w5369
                              tunnel: w5370 -> [w5374 _]
